vi "[SubVI]ENC_Read (FPGA).vi"() -> (0 "Right Theta":sgl)   [LabVIEW 2019]
uses:
  <vilib>/eio/EIONode/EIONode.xnode
  <vilib>/rvi/eio/common/nirviEmuTemplateMethod_errors.vi
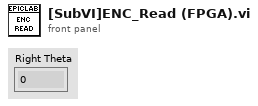
[diagram p1: front panel]
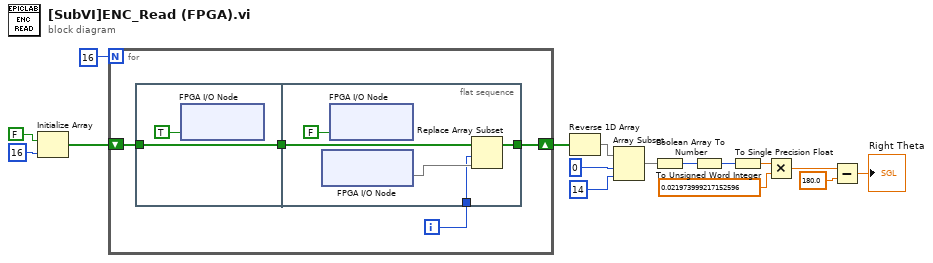
[diagram p0: block diagram]
diagram:
  n1 = Initialize Array(FALSE, 16 ("dimension size")) -> (w10:bool[])
  n2 = for {
    N: 16 -> [_]
    shift-right: [w17] -> w16
    shift-left: w10 -> [w18]
    i -> [w20]
    n3 = flat-sequence {
      tunnel: [w21] -> w19
      tunnel: w18 -> [w21]
      tunnel: w20 -> [w25]
      tunnel: w19 -> [w24]
      tunnel: [w23] -> w17
      frame #0 {
        n4 = xnode "FPGA I/O Node"("SPI.CLK"=TRUE) -> ()  [unwired: 1 in, 1 out]
      }
      frame #1 {
        n5 = xnode "FPGA I/O Node"() -> ("SPI.MISO"=w26)  [unwired: 1 in, 1 out]
        n6 = xnode "FPGA I/O Node"("SPI.CLK"=FALSE) -> ()  [unwired: 1 in, 1 out]
        n7 = Replace Array Subset(array=w24, new element=w26, index=w25) -> (w23:bool[])
      }
    }
  }
  n8 = Reverse 1D Array(array=w16) -> (reversed array=w13:bool[])
  n9 = Array Subset(array=w13, index=0, length=14) -> (w15:bool[])
  n10 = Boolean Array To Number(Boolean array=w15) -> (number=w14:u16)
  n11 = To Unsigned Word Integer(number=w14) -> (unsigned 16bit integer=w2:u16)
  n12 = To Single Precision Float(number=w2) -> (single precision float=w6:sgl)
  n13 = Multiply(x=w6, y=sgl 0.021974) -> (x*y=w3:sgl)
  n14 = Subtract(x=w3, y=sgl 180.0) -> (x-y=→"Right Theta":sgl)
